vi "Stop Stream and Reset TX FIFO.vi"(8 "error in (no error)":errorcluster, 10 "2 USRPs?":bool[](array[boolean]), 11 "Refnum in":refnum<k20>[](array[refnum])) -> (0 "error out":errorcluster, 3 "Refnum out":refnum<k20>[](array[refnum]))   [LabVIEW 2016]
uses:
  <instrlib>/_niInstr/Streaming/v1/Host/niInstr Streaming v1 Host.lvlib
  6592R/SubVIs/Aurora Stream (NI 6592R) (Host).lvlib
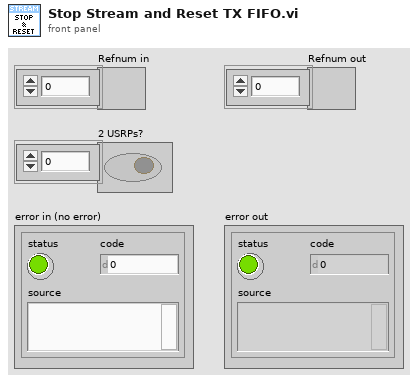
[diagram p1: front panel]
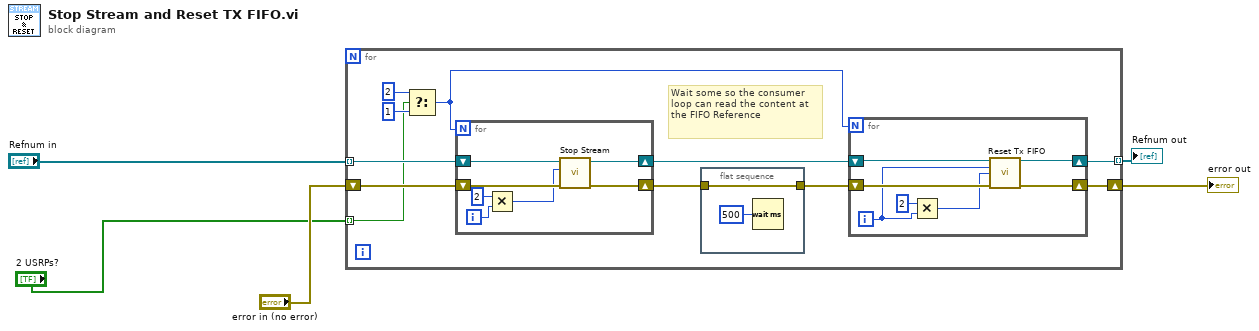
[diagram p0: block diagram]
diagram:
  n1 = for {
    tunnel: "Refnum in" -> [w15] mode=indexing
    tunnel: [w9] -> w2 mode=indexing
    shift-right: [w10] -> w3
    shift-left: "error in (no error)" -> [w16]
    tunnel: "2 USRPs?" -> [w12] mode=indexing
    # "Wait some so the consumer loop can read the content at the FIFO Reference"
    n2 = Select(t=2, s=w12, f=1) -> (s? t:f=w6:i32)
    n3 = for {
      N: w6 -> [_]
      shift-right: [w30] -> w11
      shift-left: w15 -> [w31]
      shift-right: [w29] -> w8
      shift-left: w16 -> [w32]
      i -> [w27]
      n4 = Multiply(x=2, y=w27) -> (x*y=w26:i32)
      n5 = call <instrlib>:"Stop Stream.vi"("error in (no error)"=w32, "stream index"=w26, "refnum in"=w31) -> ("error out"=w29:errorcluster, "refnum out"=w30:refnum<k20>)  [unwired: 5 in, 2 out]
    }
    n6 = flat-sequence {
      tunnel: w8 -> [w18]
      tunnel: [w18] -> w7
      frame #0 {
        n7 = Wait (ms)(milliseconds to wait=u32 500) -> ()  [unwired: 1 out]
      }
    }
    n8 = for {
      N: w6 -> [_]
      shift-right: [w23] -> w9
      shift-left: w11 -> [w24]
      shift-right: [w22] -> w10
      shift-left: w7 -> [w21]
      i -> [w19]
      n9 = Multiply(x=2, y=w19) -> (x*y=w20:i32)
      n10 = call "Reset Tx FIFO.vi"("Refnum in"=w24, "Port"=w19, "stream index"=w20, "error in"=w21) -> ("Refnum out"=w23:refnum<k20>, "error out"=w22:errorcluster)  [unwired: 10 in]
    }
  }
  "error out" <- w3
  "Refnum out" <- w2
